vi "radio_transmission_mode.vi"(8 "error in":errorcluster, 10 "message":string, 11 "VISA in":refnum<visa-resource-name>) -> (0 "error out":errorcluster, 1 "error":bool, 3 "VISA out":refnum<visa-resource-name>)   [LabVIEW 2011]
panel:
  out "read buffer 2":string
  out "read buffer 1":string
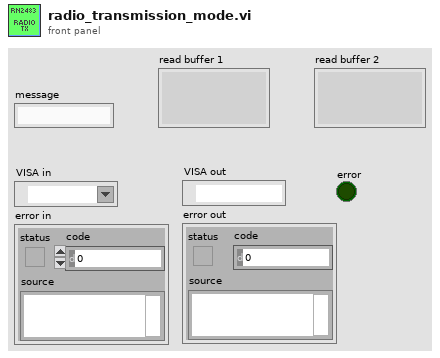
[diagram p1: front panel]
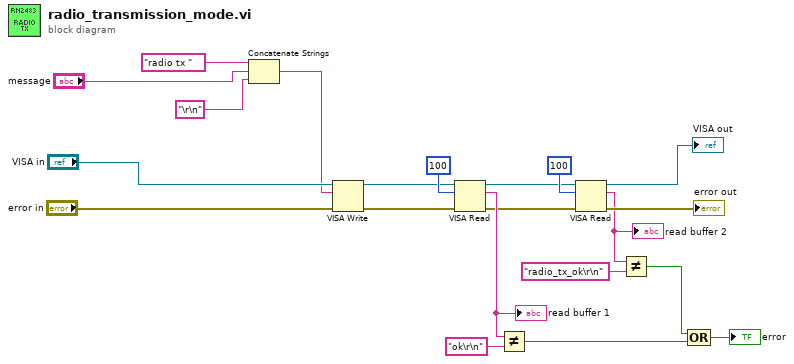
[diagram p0: block diagram]
diagram:
  n1 = Concatenate Strings("radio tx " ("string to write"), "message", "\r\n" ("string to write")) -> (w11:string)
  n2 = VISA Write(VISA resource name="VISA in", write buffer=w11, error in (no error)="error in") -> (VISA resource name out=w18:refnum<visa-resource-name>, error out=w17:errorcluster)  [unwired: 1 out]
  n3 = VISA Read(VISA resource name=w18, byte count=u32 100, error in (no error)=w17) -> (VISA resource name out=w9:refnum<visa-resource-name>, read buffer=w16:string, error out=w8:errorcluster)  [unwired: 1 out]
  "read buffer 1" <- w16
  n4 = Not Equal?(x=w16, y="ok\r\n") -> (x != y?=w4:bool)
  n5 = VISA Read(VISA resource name=w9, byte count=u32 100, error in (no error)=w8) -> (VISA resource name out=→"VISA out":refnum<visa-resource-name>, read buffer=w1:string, error out=→"error out":errorcluster)  [unwired: 1 out]
  "read buffer 2" <- w1
  n6 = Not Equal?(x=w1, y="radio_tx_ok\r\n") -> (x != y?=w2:bool)
  n7 = Compound Arithmetic op=OR(w2, w4) -> (→"error":bool)
